vi "T_CH-Main.vi"() -> ()   [LabVIEW 2021]
doc: "Use this template to build a simple state machine design pattern. Each state executes code and determines which state to transition to."
uses:
  controls/MainData.ctl
  controls/MainState.ctl
  <instrlib>/Keithley 2450/Keithley 2450.lvlib
panel:
  in  "rearm delay":u32=200
  in  "reading delay":u32=6000
  in  "VISA Gate SMU":refnum<visa-resource-name>="USB0::0x05E6::0x2450::04408955::INSTR"
  in  "VISA Drain SMU":refnum<visa-resource-name>="USB0::0x05E6::0x2450::04405250::INSTR"
  out "Data":T1={"Measurement running"=FALSE, "Info message"="Exiting app.", "Drain Voltage (V)"=[], "Drain current (A)"=[], "Gate voltage (V)"=[], "Gate current (A)"=[], "Drain SMU"="USB0::0x05E6::0x2450::04405250::INSTR", "Gate SMU"="USB0::0x05E6::0x2450::04408955::INSTR", "Gate index"=6, "tdms file path"=path ""}
  in  "Gate sweep":T2={"Start (V) "=-5.0, "Stop( V) "=5.0, "Points (-)"=6, "Delay (s)"=0.01, "Limit  Level (A)"=0.1} {"Limit  Level (A)" format="%#_13g"; "Delay (s)" format="%#_13g"}
  out "XY Graph":cluster{dbl[], dbl[]}(graph)
  in  "Drain sweep":T2={"Start (V) "=0.0, "Stop( V) "=0.5, "Points (-)"=30, "Delay (s)"=0.01, "Limit  Level (A)"=0.1} {"Limit  Level (A)" format="%#_13g"; "Delay (s)" format="%#_13g"}
  in  "Stop measurement":bool
  in  "Start measurement":bool
  in  "Exit":bool
  # "about 6 seconds per 30 points"
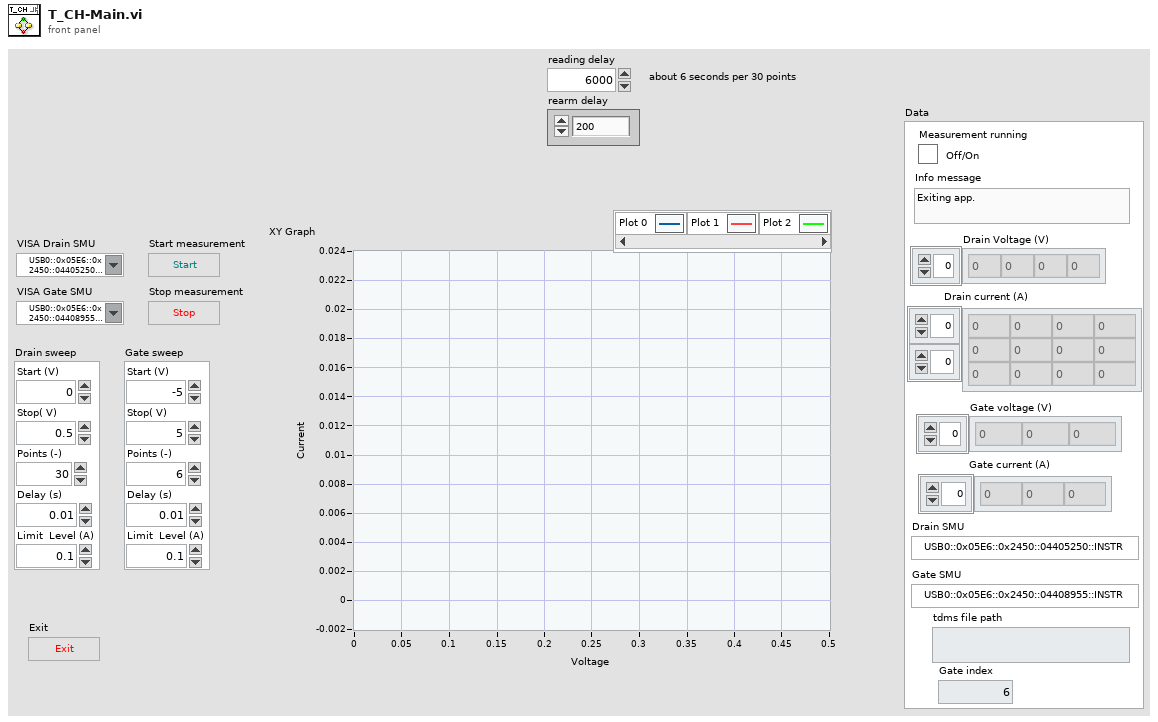
[diagram p1: front panel]
types:
  T1 = typedef "MainData.ctl" = cluster{"Measurement running":bool, "Info message":string, "Drain Voltage (V)":dbl[], "Drain current (A)":dbl[][], "Gate voltage (V)":dbl[], "Gate current (A)":dbl[], "Drain SMU":refnum<visa-resource-name>, "Gate SMU":refnum<visa-resource-name>, "Gate index":u32, "tdms file path":path}
  T2 = cluster{"Start (V) ":dbl, "Stop( V) ":dbl, "Points (-)":u32, "Delay (s)":dbl, "Limit  Level (A)":dbl}
  T3 = typedef "MainState.ctl" = enum16{"Initialize", "Wait for Event", "START measurement", "Connect SMUs", "Setup measurement", "Step gate voltage", "Read gate current", "Sweep drain voltage", "Check drain current", "Next step", "STOP measurement", "Disconnect SMUs", "EXIT app"}
  T4 = enum16{"open", "open or create", "create or replace", "create", "open (read-only)"}
  T5 = cluster{"Drain Voltage (V)":dbl[], "Current":dbl[]}
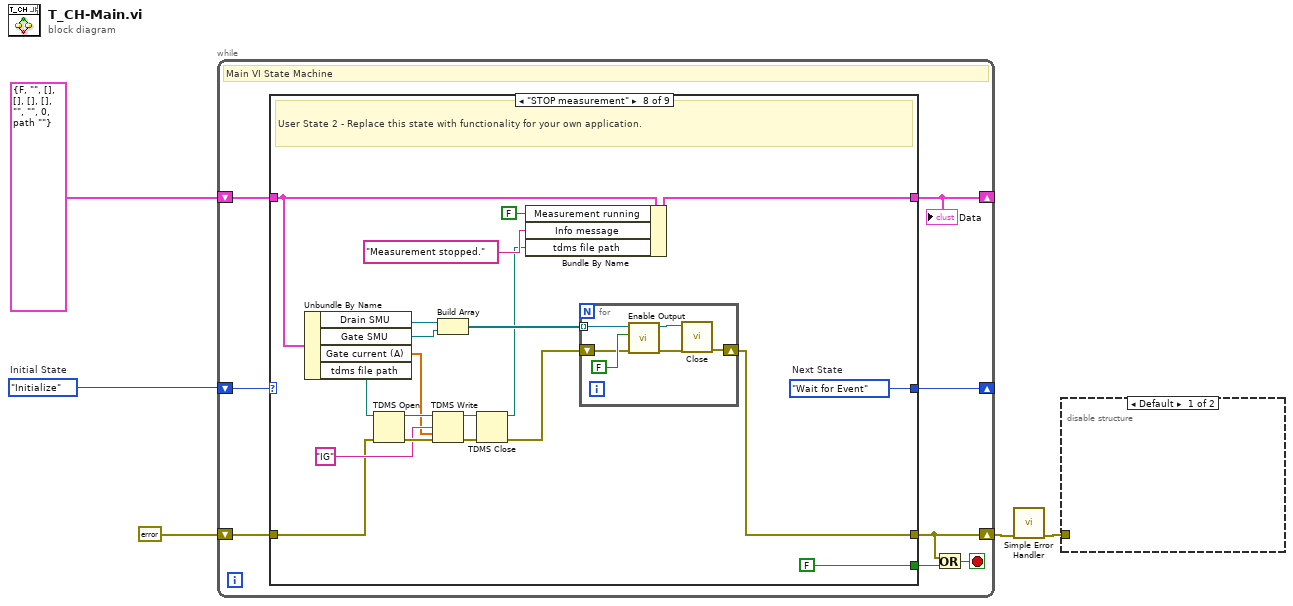
[diagram p0: block diagram]
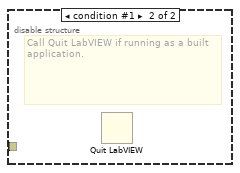
[diagram p2: hidden frame]
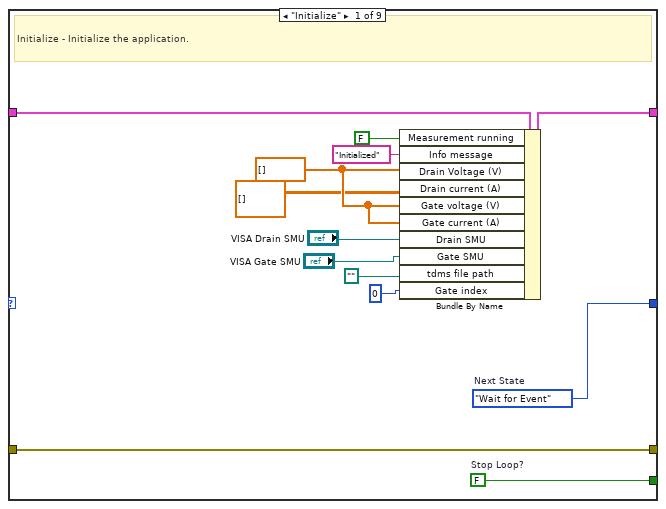
[diagram p3: hidden frame]
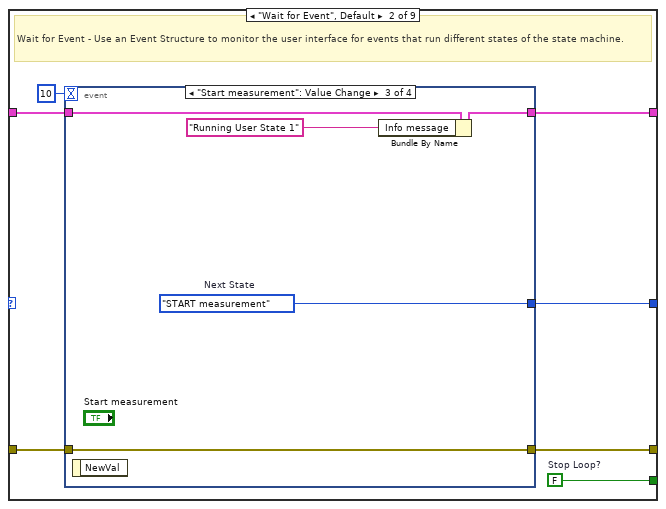
[diagram p4: hidden frame]
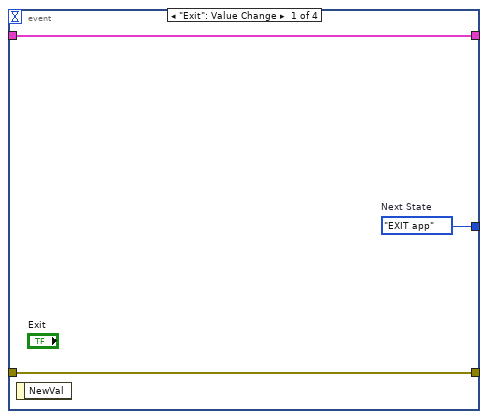
[diagram p5: hidden frame]
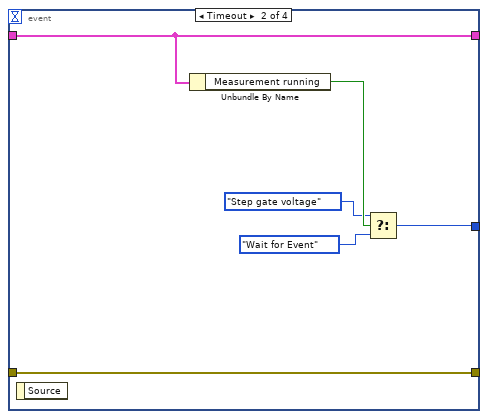
[diagram p6: hidden frame]
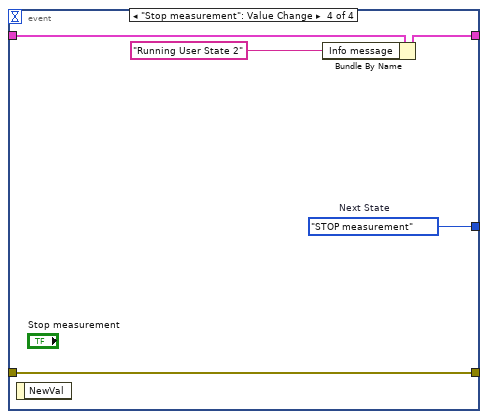
[diagram p7: hidden frame]
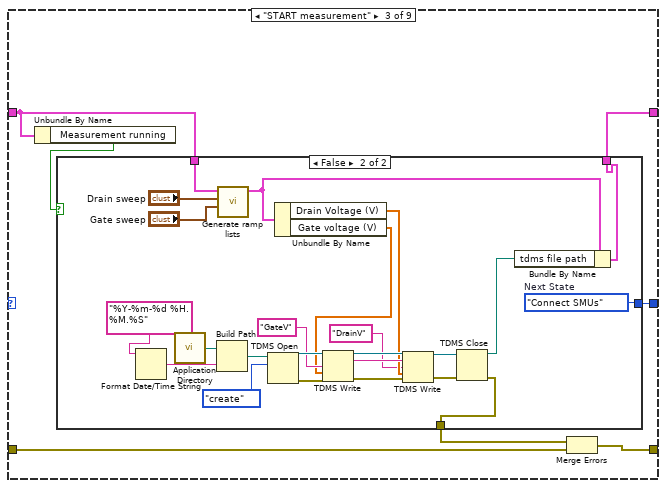
[diagram p8: hidden frame]
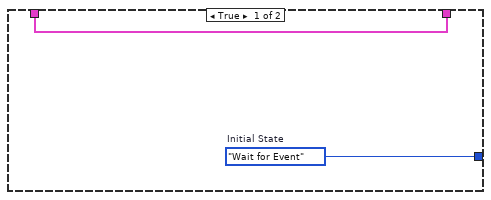
[diagram p9: hidden frame]
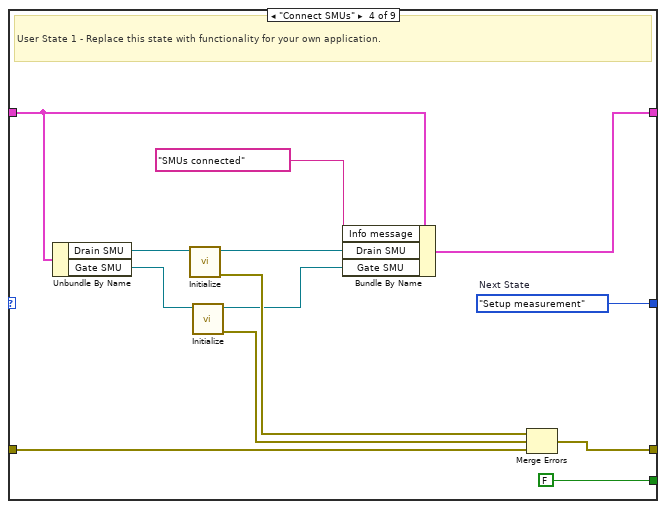
[diagram p10: hidden frame]
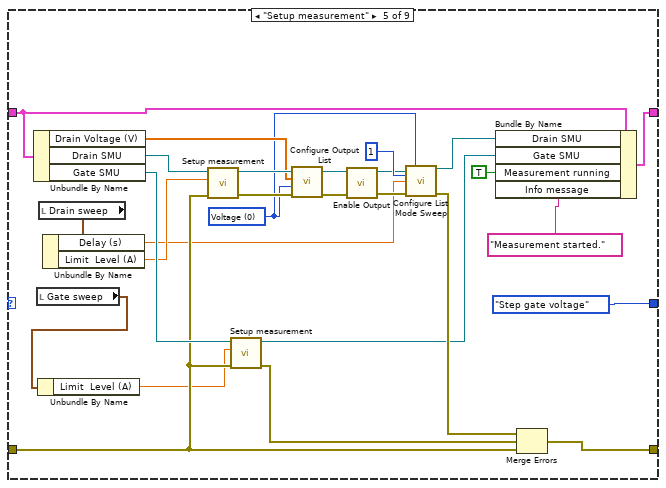
[diagram p11: hidden frame]
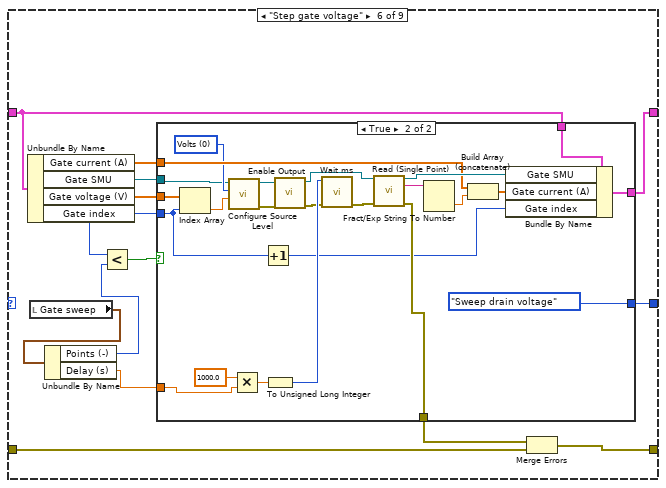
[diagram p12: hidden frame]
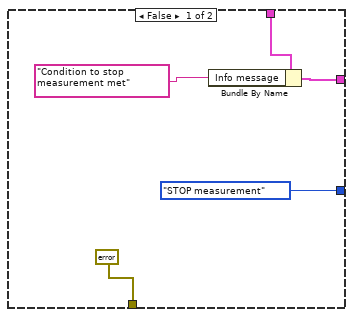
[diagram p13: hidden frame]
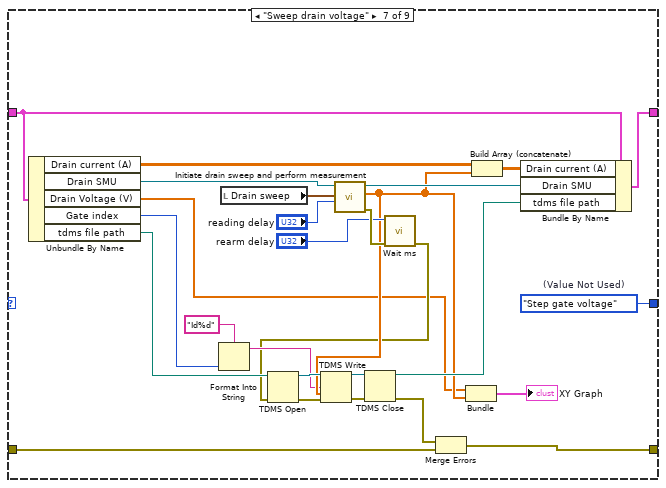
[diagram p14: hidden frame]
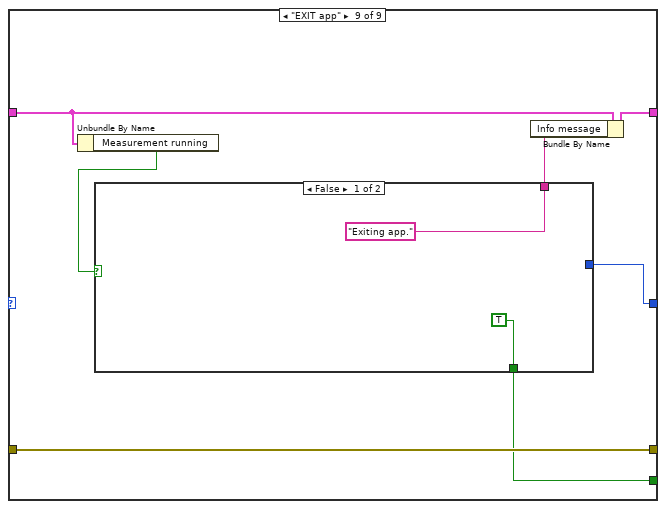
[diagram p15: hidden frame]
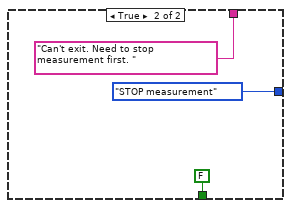
[diagram p16: hidden frame]
diagram:
  w5 = MainState."Initialize"  # Initial State
  n1 = while {
    shift-right: [w12] -> _
    shift-left: w5 -> [w13]
    shift-right: [w10] -> _
    shift-left: T1 {"Measurement running"=FALSE, "Info message"="", "Drain Voltage (V)"=[], "Drain current (A)"=[], "Gate voltage (V)"=[], "Gate current (A)"=[], "Drain SMU"="", "Gate SMU"="", "Gate index"=0, "tdms file path"=path ""} ("Data") -> [w11]
    shift-right: [w6] -> w2
    shift-left: errorcluster {"status"=FALSE, "code"=0, "source"=""} ("error constant") -> [w9]
    stop <- w7 stop-if-true
    # "Main VI State Machine"
    n2 = case shown="\"STOP measurement\"" w13 {
      tunnel: [w26 w33 w57 w98 MainState."Step gate voltage" ("Next State") w138 w186 w215 w227] -> w12
      tunnel: [w25 w32 _ FALSE ("Stop Loop?") _ _ _ FALSE ("Stop Loop?") w224] -> w8
      tunnel: w11 -> [w24 w31 w56 w96 w124 w131 w194 w213 w226]
      tunnel: [w23 w30 w55 w89 w106 w130 w192 w208 w223] -> w10
      tunnel: w9 -> [w21 w29 w59 w94 w121 w139 w172 w196 w228]
      tunnel: [w21 w28 w54 w93 w120 w128 w188 w209 w228] -> w6
      frame "Initialize" {
        w19 = dbl[] [] ("Drain Voltage (V)")
        w25 = FALSE  # Stop Loop?
        w26 = MainState."Wait for Event"  # Next State
        # "Initialize - Initialize the application."
        n3 = Bundle By Name(cluster=w24, "Measurement running"=FALSE ("Replace_Me_Boolean"), "Info message"="Initialized" ("Stage"), "Drain Voltage (V)"=w19, "Drain current (A)"=dbl[][] [], "Gate voltage (V)"=w19, "Gate current (A)"=w19, "Drain SMU"="VISA Drain SMU", "Gate SMU"="VISA Gate SMU", "tdms file path"=path "", "Gate index"=0 ("Drain index")) -> (w23:T1)
      }
      frame "Wait for Event", Default {
        w32 = FALSE  # Stop Loop?
        # "Wait for Event - Use an Event Structure to monitor the user interface for events that run different states of the state machine."
        n4 = event shown="[2] \"Start measurement\": Value Change" {
          selector: _ -> [_ _ _ _]
          dyn-events: _ -> [_ _ _ _]
          timeout: 10 -> [_ _ _ _]
          tunnel: [w36 w37 w47 w52] -> w33
          tunnel: w31 -> [w35 w41 w46 w51]
          tunnel: [w35 w41 w45 w50] -> w30
          tunnel: w29 -> [w34 w42 w43 w48]
          tunnel: [w34 w42 w43 w48] -> w28
          event "Exit": Value Change {
            w36 = MainState."EXIT app"  # Next State
            n5 = event-data() -> ()  [unwired: 1 in, 1 out]
          }
          event Timeout {
            n6 = event-data() -> ()  [unwired: 1 in, 1 out]
            n7 = Unbundle By Name(w41) -> ("Measurement running"=w40:bool)
            n8 = Select(t=MainState."Step gate voltage", s=w40, f=MainState."Wait for Event" ("Next State")) -> (s? t:f=w37:T3)
          }
          event "Start measurement": Value Change {
            w47 = MainState."START measurement"  # Next State
            n9 = event-data() -> ()  [unwired: 1 in, 1 out]
            n10 = Bundle By Name(cluster=w46, "Info message"="Running User State 1" ("Running User State 1")) -> (w45:T1)
          }
          event "Stop measurement": Value Change {
            w52 = MainState."STOP measurement"  # Next State
            n11 = event-data() -> ()  [unwired: 1 in, 1 out]
            n12 = Bundle By Name(cluster=w51, "Info message"="Running User State 2" ("Running User State 2")) -> (w50:T1)
          }
        }
      }
      frame "START measurement" {
        n13 = Unbundle By Name(w56) -> ("Measurement running"=w58:bool)
        n14 = case shown="False" w58 {
          tunnel: [w61 w85] -> w57
          tunnel: w56 -> [w60 w83]
          tunnel: [w60 w71] -> w55
          tunnel: [_ w62] -> w53
          frame True {
            w61 = MainState."Wait for Event"  # Initial State
          }
          frame False {
            w85 = MainState."Connect SMUs"  # Next State
            n15 = Format Date/Time String(time format string (%c)="%Y-%m-%d %H.%M.%S") -> (date/time string=w77:string)  [unwired: 2 in]
            n16 = call <vilib>:"Application Directory.vi"() -> ("Application Directory"=w79:path)
            n17 = Build Path(base path=w79, name or relative path=w77) -> (appended path=w80:path)
            n18 = call "Generate ramp lists.vi"("SMU2 settings"="Gate sweep", "SMU1 settings"="Drain sweep", "Data in"=w83) -> ("Data out"=w70:T1)  [unwired: 8 in]
            n19 = TDMS Open(10:T4."create" ("operation (0:open)"), 11:w80) -> (0:w76:errorcluster, 3:w72:refnum<k34>)  [unwired: 5 in]
            n20 = Unbundle By Name(w70) -> ("Drain Voltage (V)"=w68:dbl[], "Gate voltage (V)"=w67:dbl[])
            n21 = TDMS Write(0:w72, 7:"GateV" ("channel name(s) in (Untitled)"), 9:w67, 11:w76) -> (4:w75:refnum<k34>, 6:w74:string, 15:w73:errorcluster)  [unwired: 2 in, 1 out]
            n22 = TDMS Write(0:w75, 5:w74, 7:"DrainV" ("channel name(s) in (Untitled)"), 9:w68, 11:w73) -> (4:w65:refnum<k34>, 15:w63:errorcluster)  [unwired: 1 in, 2 out]
            n23 = TDMS Close(8:w63, 11:w65) -> (0:w62:errorcluster, 3:w64:path)
            n24 = Bundle By Name(cluster=w70, "tdms file path"=w64) -> (w71:T1)
          }
        }
        n25 = Merge Errors(w53, w59) -> (w54:errorcluster)
      }
      frame "Connect SMUs" {
        w98 = MainState."Setup measurement"  # Next State
        # "User State 1 - Replace this state with functionality for your own application."
        n26 = Unbundle By Name(w96) -> ("Drain SMU"=w95:refnum<visa-resource-name>, "Gate SMU"=w92:refnum<visa-resource-name>)
        n27 = call <instrlib>:"Initialize.vi"("VISA resource name"=w95) -> ("error out"=w90:errorcluster, "VISA resource name out"=w88:refnum<visa-resource-name>)  [unwired: 9 in]
        n28 = call <instrlib>:"Initialize.vi"("VISA resource name"=w92) -> ("error out"=w91:errorcluster, "VISA resource name out"=w87:refnum<visa-resource-name>)  [unwired: 9 in]
        n29 = Bundle By Name(cluster=w96, "Info message"="SMUs connected", "Drain SMU"=w88, "Gate SMU"=w87) -> (w89:T1)
        n30 = Merge Errors(w90, w91, w94) -> (w93:errorcluster)
      }
      frame "Setup measurement" {
        w99 = u16 0 items=["Voltage", "Current"] ("Source Mode  (0: Voltage)")
        n31 = Unbundle By Name(w124) -> ("Drain Voltage (V)"=w112:dbl[], "Drain SMU"=w123:refnum<visa-resource-name>, "Gate SMU"=w122:refnum<visa-resource-name>)
        n32 = local read "Gate sweep"() -> (w103:T2)
        n33 = Unbundle By Name(w103) -> ("Limit  Level (A)"=w102:dbl)
        n34 = local read "Drain sweep"() -> (w111:T2)
        n35 = Unbundle By Name(w111) -> ("Delay (s)"=w109:dbl, "Limit  Level (A)"=w110:dbl)
        n36 = call "Setup measurement.vi"("error in (no error)"=w121, "Source Limit Level (0.1)"=w110, "VISA Refnum in"=w123) -> ("error in (no error) 2"=w113:errorcluster, "VISA resource name out"=w114:refnum<visa-resource-name>)  [unwired: 7 in]
        n37 = call "Setup measurement.vi"("error in (no error)"=w121, "Source Limit Level (0.1)"=w102, "VISA Refnum in"=w122) -> ("error in (no error) 2"=w107:errorcluster, "VISA resource name out"=w104:refnum<visa-resource-name>)  [unwired: 7 in]
        n38 = call <instrlib>:"Configure Output List.vi"("error in (no error)"=w113, "Source Mode  (0: Voltage)"=w99, "Output List"=w112, "VISA resource name"=w114) -> ("error out"=w119:errorcluster, "VISA resource name out"=w115:refnum<visa-resource-name>)  [unwired: 6 in]
        n39 = call <instrlib>:"Enable Output.vi"("error in (no error)"=w119, "VISA resource name"=w115) -> ("error out"=w118:errorcluster, "VISA resource name out"=w116:refnum<visa-resource-name>)  [unwired: 8 in]
        n40 = call <instrlib>:"Configure List Mode Sweep.vi"("VISA resource name"=w116, "Source Mode  (0: Voltage)"=w99, "Start Index"=u32 1, "Delay (0)"=w109, "error in (no error)"=w118) -> ("VISA resource name out"=w105:refnum<visa-resource-name>, "error out"=w108:errorcluster)  [unwired: 9 in]
        n41 = Bundle By Name(cluster=w124, "Drain SMU"=w105, "Gate SMU"=w104, "Measurement running"=TRUE, "Info message"="Measurement started.") -> (w106:T1)
        n42 = Merge Errors(w108, w107, w121) -> (w120:errorcluster)
      }
      frame "Step gate voltage" {
        n43 = Unbundle By Name(w131) -> ("Gate current (A)"=w126:dbl[], "Gate SMU"=w137:refnum<visa-resource-name>, "Gate voltage (V)"=w133:dbl[], "Gate index"=w132:u32)
        n44 = local read "Gate sweep"() -> (w135:T2)
        n45 = Unbundle By Name(w135) -> ("Points (-)"=w134:u32, "Delay (s)"=w129:dbl)
        n46 = Less?(x=w132, y=w134) -> (x < y?=w136:bool)
        n47 = case shown="True" w136 {
          tunnel: [MainState."STOP measurement" ("Next State") MainState."Sweep drain voltage" ("Next State")] -> w138
          tunnel: w137 -> [_ w150]
          tunnel: w133 -> [_ w167]
          tunnel: w132 -> [_ w146]
          tunnel: w131 -> [w143 w166]
          tunnel: [w141 w165] -> w130
          tunnel: w129 -> [_ w164]
          tunnel: [errorcluster {"status"=FALSE, "code"=0, "source"=""} ("error in (no error) 2") w148] -> w127
          tunnel: w126 -> [_ w156]
          frame False {
            n48 = Bundle By Name(cluster=w143, "Info message"="Condition to stop measurement met") -> (w141:T1)
          }
          frame True {
            w152 = u16 0 items=["Volts", "Current"] ("Function (0: Volts)")
            n49 = Index Array(array=w167, index=w146) -> (element=w151:dbl)
            n50 = call <instrlib>:"Configure Source Level.vi"("Source Level (1.0)"=w151, "Function (0: Volts)"=w152, "VISA resource name"=w150) -> ("error out"=w153:errorcluster, "VISA resource name out"=w149:refnum<visa-resource-name>)  [unwired: 7 in]
            n51 = Multiply(x=1000.0, y=w164) -> (x*y=w163:dbl)
            n52 = Increment(x=w146) -> (x+1=w145:u32)
            n53 = To Unsigned Long Integer(number=w163) -> (unsigned 32bit integer=w161:u32)
            n54 = call <instrlib>:"Enable Output.vi"("error in (no error)"=w153, "VISA resource name"=w149) -> ("error out"=w160:errorcluster, "VISA resource name out"=w159:refnum<visa-resource-name>)  [unwired: 8 in]
            n55 = call "Wait ms.vi"("error in (no error)"=w160, "milliseconds to wait"=w161) -> ("error in (no error) 2"=w158:errorcluster)  [unwired: 9 in]
            n56 = call <instrlib>:"Read (Single Point).vi"("VISA resource name"=w159, "error in (no error)"=w158) -> ("VISA resource name out"=w157:refnum<visa-resource-name>, "Data out"=w154:string, "error out"=w148:errorcluster)  [unwired: 11 in]
            n57 = Fract/Exp String To Number(string=w154) -> (number=w147:dbl)  [unwired: 3 in, 1 out]
            n58 = Build Array (concatenate)(w156, w147) -> (w155:dbl[])
            n59 = Bundle By Name(cluster=w166, "Gate SMU"=w157, "Gate current (A)"=w155, "Gate index"=w145) -> (w165:T1)
          }
        }
        n60 = Merge Errors(w127, w139) -> (w128:errorcluster)
      }
      frame "Sweep drain voltage" {
        w186 = MainState."Step gate voltage"  # (Value Not Used)
        n61 = Unbundle By Name(w194) -> ("Drain current (A)"=w190:dbl[][], "Drain SMU"=w193:refnum<visa-resource-name>, "Drain Voltage (V)"=w169:dbl[], "Gate index"=w175:u32, "tdms file path"=w182:path)
        n62 = Format Into String(format string="Id%d", w175) -> (resulting string=w173:string)  [unwired: 2 in, 1 out]
        n63 = local read "Drain sweep"() -> (w195:T2)
        n64 = call "Initiate drain sweep and perform measurement.vi"("reading delay"="reading delay", "Drain sweep"=w195, "VISA Refnum in"=w193) -> ("error out"=w185:errorcluster, "Current"=w176:dbl[], "VISA Refnum out"=w191:refnum<visa-resource-name>)  [unwired: 6 in]
        n65 = call "Wait ms.vi"("error in (no error)"=w185, "milliseconds to wait"="rearm delay") -> ("error in (no error) 2"=w170:errorcluster)  [unwired: 9 in]
        n66 = TDMS Open(8:w170, 11:w182) -> (0:w177:errorcluster, 3:w181:refnum<k34>)  [unwired: 5 in]
        n67 = TDMS Write(0:w181, 7:w173, 9:w176, 11:w177) -> (4:w180:refnum<k34>, 15:w178:errorcluster)  [unwired: 2 in, 2 out]
        n68 = TDMS Close(8:w178, 11:w180) -> (0:w171:errorcluster, 3:w179:path)
        n69 = Merge Errors(w171, w172) -> (w188:errorcluster)
        n70 = Bundle("Drain Voltage (V)"=w169, "Current"=w176) -> (→"XY Graph":T5)  [unwired: 1 in]
        n71 = Build Array (concatenate)(w190, w176) -> (w189:dbl[][])
        n72 = Bundle By Name(cluster=w194, "Drain current (A)"=w189, "Drain SMU"=w191, "tdms file path"=w179) -> (w192:T1)
      }
      frame "STOP measurement" {
        w215 = MainState."Wait for Event"  # Next State
        # "User State 2 - Replace this state with functionality for your own application."
        n73 = Unbundle By Name(w213) -> ("Drain SMU"=w212:refnum<visa-resource-name>, "Gate SMU"=w210:refnum<visa-resource-name>, "Gate current (A)"=w198:dbl[], "tdms file path"=w199:path)
        n74 = TDMS Open(8:w196, 11:w199) -> (0:w204:errorcluster, 3:w205:refnum<k34>)  [unwired: 5 in]
        n75 = TDMS Write(0:w205, 7:"IG" ("format string"), 9:w198, 11:w204) -> (4:w203:refnum<k34>, 15:w202:errorcluster)  [unwired: 2 in, 2 out]
        n76 = Build Array(w212, w210) -> (w211:refnum<visa-resource-name>[])
        n77 = TDMS Close(8:w202, 11:w203) -> (0:w200:errorcluster, 3:w197:path)
        n78 = Bundle By Name(cluster=w213, "Measurement running"=FALSE, "Info message"="Measurement stopped.", "tdms file path"=w197) -> (w208:T1)
        n79 = for {
          tunnel: w211 -> [w221] mode=indexing
          shift-right: [w217] -> w209
          shift-left: w200 -> [w216]
          n80 = call <instrlib>:"Enable Output.vi"("error in (no error)"=w216, "Enable Output (T: Enable)"=FALSE, "VISA resource name"=w221) -> ("error out"=w218:errorcluster, "VISA resource name out"=w220:refnum<visa-resource-name>)  [unwired: 7 in]
          n81 = call <instrlib>:"Close.vi"("error in (no error)"=w218, "VISA resource name"=w220) -> ("error out"=w217:errorcluster)  [unwired: 9 in]
        }
      }
      frame "EXIT app" {
        n82 = Unbundle By Name(w226) -> ("Measurement running"=w225:bool)
        n83 = case shown="False" w225 {
          tunnel: [_ MainState."STOP measurement" ("t")] -> w227
          tunnel: [TRUE FALSE] -> w224
          tunnel: ["Exiting app." "Can't exit. Need to stop measurement first. "] -> w222
          frame False {
          }
          frame True {
          }
        }
        n84 = Bundle By Name(cluster=w226, "Info message"=w222) -> (w223:T1)
      }
    }
    "Data" <- w10
    n85 = Or(x=w6, y=w8) -> (x .or. y?=w7:bool)
  }
  n86 = call <vilib>:"Simple Error Handler.vi"("error in (no error)"=w2) -> ("error out"=w1:errorcluster)  [unwired: 4 in, 4 out]
  n87 = disable-structure shown="Default" {
    disable-tunnel: w1 -> [_ _]
    frame condition #0 (active) {
    }
    frame condition #1 {
      # "Call Quit LabVIEW if running as a built application."
      n88 = Quit LabVIEW() -> ()  [unwired: 1 in]
    }
  }
